vi "HIOKI PW3390 IDN.vi"(8 "error in (no error)":errorcluster, 11 "VISA Resource":refnum<visa-resource-name>) -> (0 "error out":errorcluster, 2 "ID":string, 3 "VISA Resource out":refnum<visa-resource-name>)   [LabVIEW 2009]
doc: "Queries the Device ID.\n\n<B>Note</B>\nOutput Items:<Maker>, <Model>, <Serial Number>, <Software Version>\nExamples: HIOKI,PW3390-03,****,V1.00"
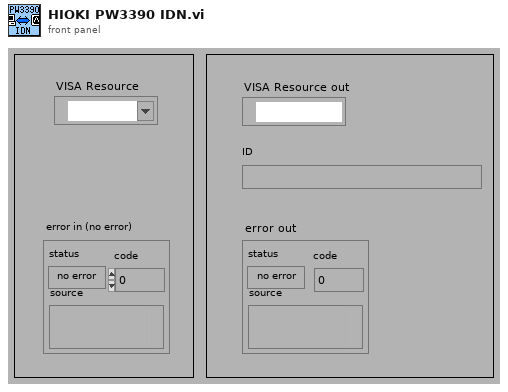
[diagram p1: front panel]
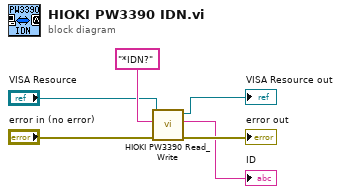
[diagram p0: block diagram]
diagram:
  n1 = call <instrlib>:"HIOKI PW3390 Read_Write.vi"("error in (no error)"="error in (no error)", "data in"="*IDN?", "VISA Resource"="VISA Resource") -> ("error out"=→"error out":errorcluster, "data out"=→"ID":string, "VISA Resource out"=→"VISA Resource out":refnum<visa-resource-name>)  [unwired: 6 in]
